vi "Z Go.vi"(8 "error in (no error)":errorcluster, 9 "Speed":dbl format="%#_13g", 10 "Position":dbl format="%#_13g", 11 "Gantry in":refnum<class "A3200.lvclass">) -> (0 "error out":errorcluster, 3 "Gantry out":refnum<class "A3200.lvclass">)   [LabVIEW 2016, in "A3200.lvclass"]
uses:
  A3200.lvclass
  A3200.lvclass/A3200.ctl
  Drivers/Aerotech A3200/Aerotech VIs.lvlib
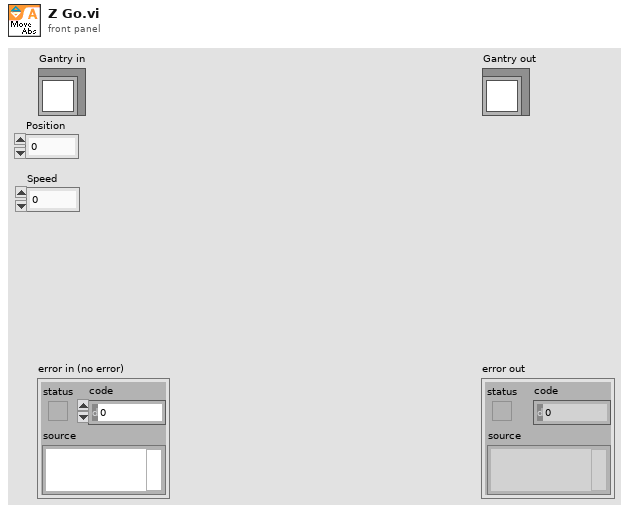
[diagram p1: front panel]
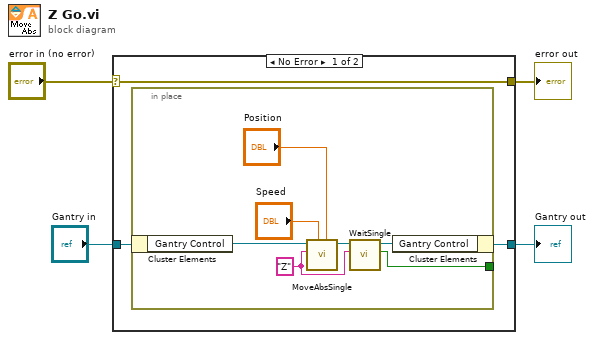
[diagram p0: block diagram]
diagram:
  n1 = case shown="No Error" "error in (no error)" {
    selector: "error in (no error)" -> [w5 w16]
    tunnel: "Gantry in" -> [w7 w15]
    tunnel: [w6 w15] -> w3
    tunnel: [w5 w16] -> w1
    frame No Error {
      n2 = in-place {
        in-place-border: [w9] -> _
        w8 = "Z"
        n3 = in-place-cluster #1(w7) -> ("Gantry Control"=w14:refnum<k24>)
        n4 = call "MoveAbsSingle.vi"("position"="Position", "speed"="Speed", "axis name"=w8, "controller in"=w14) -> ("controller out"=w12:refnum<k24>)  [unwired: 6 in, 1 out]
        n5 = call "WaitSingle.vi"("axis name"=w8, "controller in"=w12) -> ("completed"=w9:bool, "controller out"=w13:refnum<k24>)  [unwired: 7 in, 1 out]
        n6 = in-place-cluster #1("Gantry Control"=w13) -> (w6:refnum<class "A3200.lvclass">)
      }
    }
    frame Error {
    }
  }
  "error out" <- w1
  "Gantry out" <- w3
